vi "SizeofArray.vi"() -> ()   [LabVIEW 2019]
panel:
  out "size(s) 2":i32[](array[numeric])
  in  "aStr2D":string[][](array[string])
  out "size(s)":i32
  in  "aStr":string[](array[string])
  # "Row"
  # "Col"
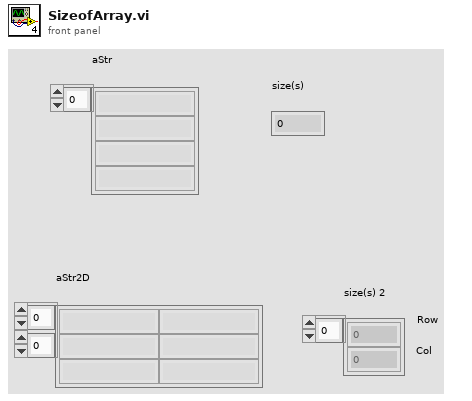
[diagram p1: front panel]
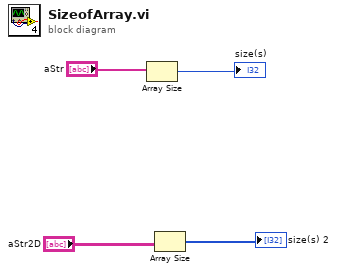
[diagram p0: block diagram]
diagram:
  n1 = Array Size(array="aStr") -> (size(s)=→"size(s)":i32)
  n2 = Array Size(array="aStr2D") -> (size(s)=→"size(s) 2":i32[])
